vi "Remove invalid characters.vi"(11 "String in":string) -> (3 "result string":string)   [LabVIEW 2020]
doc: "Removes characters that are invalid from a string."
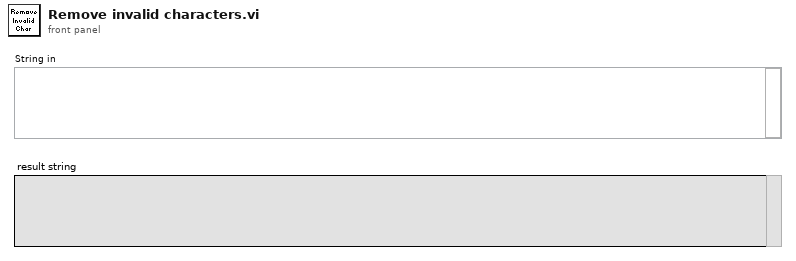
[diagram p1: front panel]
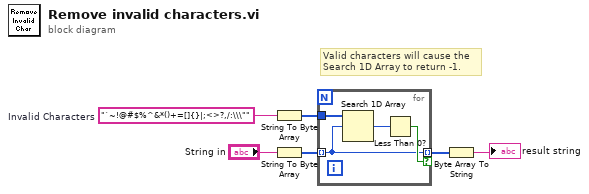
[diagram p0: block diagram]
diagram:
  w1 = "`~!@#$%^&*()+=[]{}|;<>?,/:\\\""  # Invalid Characters
  # "Valid characters will cause the \nSearch 1D Array to return -1."
  n1 = String To Byte Array(string=w1) -> (unsigned byte array=w6:u8[])
  n2 = String To Byte Array(string="String in") -> (unsigned byte array=w5:u8[])
  n3 = for {
    tunnel: w5 -> [w7] mode=indexing
    tunnel: w6 -> [w10]
    tunnel: [w7] -> w4 mode=indexing if=w8
    n4 = Search 1D Array(1D array=w10, element=w7) -> (index of element=w9:i32)  [unwired: 1 in]
    n5 = Less Than 0?(x=w9) -> (x < 0?=w8:bool)
  }
  n6 = Byte Array To String(unsigned byte array=w4) -> (string=→"result string":string)
